vi "Client.vi"() -> ()   [LabVIEW 2018]
uses:
  <vilib>/Utility/error.llb/DialogType.ctl
  <vilib>/Utility/file.llb/Write Delimited Spreadsheet (string).vi
panel:
  in  "Address/IP":string="localhost"
  in  "Remote port or service name":u16=6340
  in  "Start":bool
  in  "file path (dialog if empty)":path=path "C:/Users/Sagar/Desktop/MEE 5318/Project4/data.txt"
  out "Waveform Graph":waveform(dbl)(graph)
  out "ai0 X-axis Waveform Graph":waveform(dbl)[](graph)
  out "ai1 Y-axis Waveform Graph":waveform(dbl)[](graph)
  out "appended array 2":dbl[][](array[numeric])
  in  "appended array":dbl[][](array[numeric])
  in  "Number of Samples":dbl=2000.0
  in  "Sample Rate":dbl=1000.0
  in  "Counter":tag="myDAQ1/ctr0"
  in  "Analog Physical Channel 1":tag="myDAQ1/ai0"
  in  "Analog Physical Channel 2":tag="myDAQ1/ai1"
  in  "IIR filter specifications":T1={"Topology"=enum."Butterworth", "Type"=enum."Lowpass", "Order"=3, "Lower Fc"=100.0, "Upper Fc"=200.0, "PB Ripple"=1.0, "SB Attenuation"=60.0} {"PB Ripple" format="%0.2f"; "SB Attenuation" format="%0.2f"; "Lower Fc" format="%0.2p"; "Upper Fc" format="%0.2p"}
  # "MEE 5318 Project 4 Client.vi\nGroup: 7\nMembers: Sagar Jagtap (903935334)\n                   Arunkumar Ramachandran (903928488)"
  # "Input following parameters and click \"START ACQUISITION\" to start acquiring data"
  # "The following graphs illustrate the acquired data"
  # "Comm Settings"
  # "Channel Settings"
  # "Timing Settings"
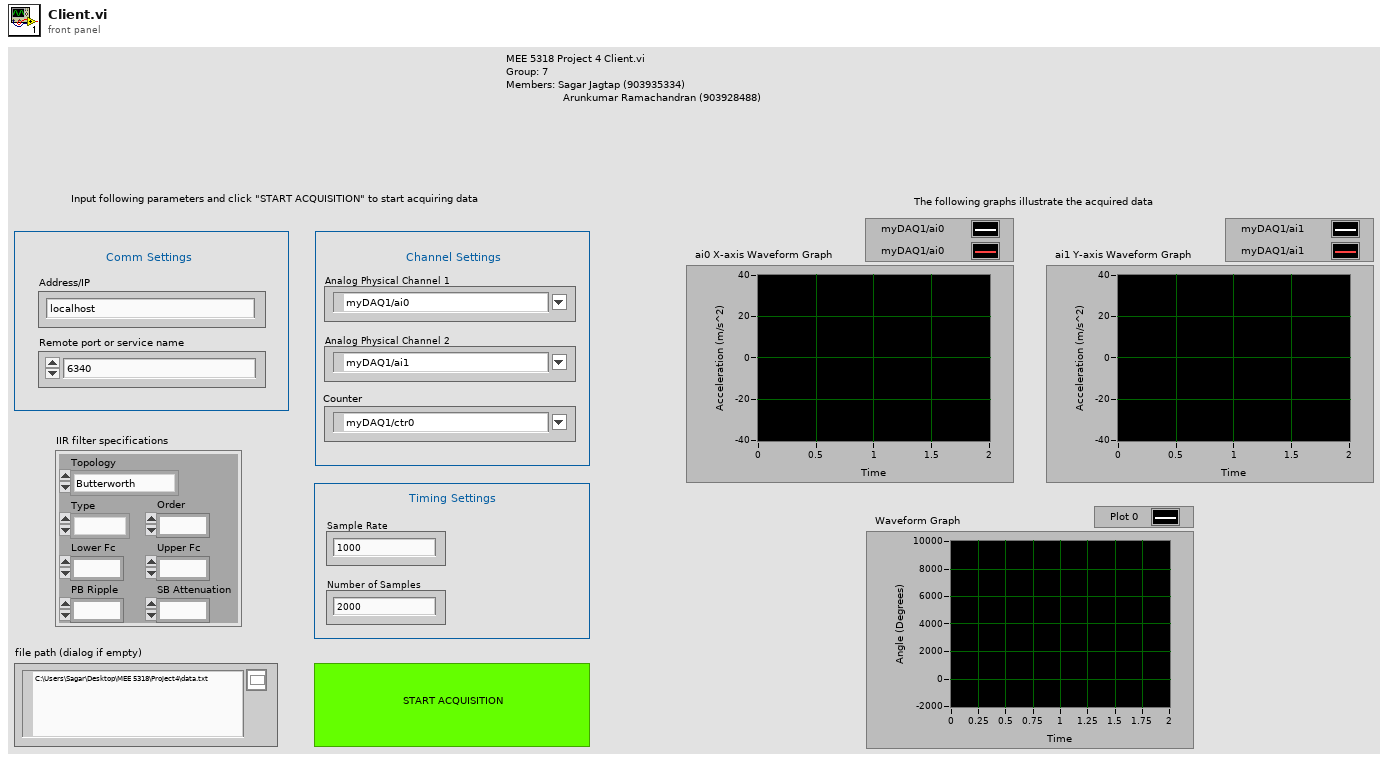
[diagram p1: front panel]
types:
  T1 = cluster{"Topology":enum16{"Off", "Butterworth", "Chebyshev", "Inverse Chebyshev", "Elliptic", "Bessel"}, "Type":enum16{"Lowpass", "Highpass", "Bandpass", "Bandstop"}, "Order":i32, "Lower Fc":dbl, "Upper Fc":dbl, "PB Ripple":dbl, "SB Attenuation":dbl}
  T2 = typedef "DialogType.ctl" = u16
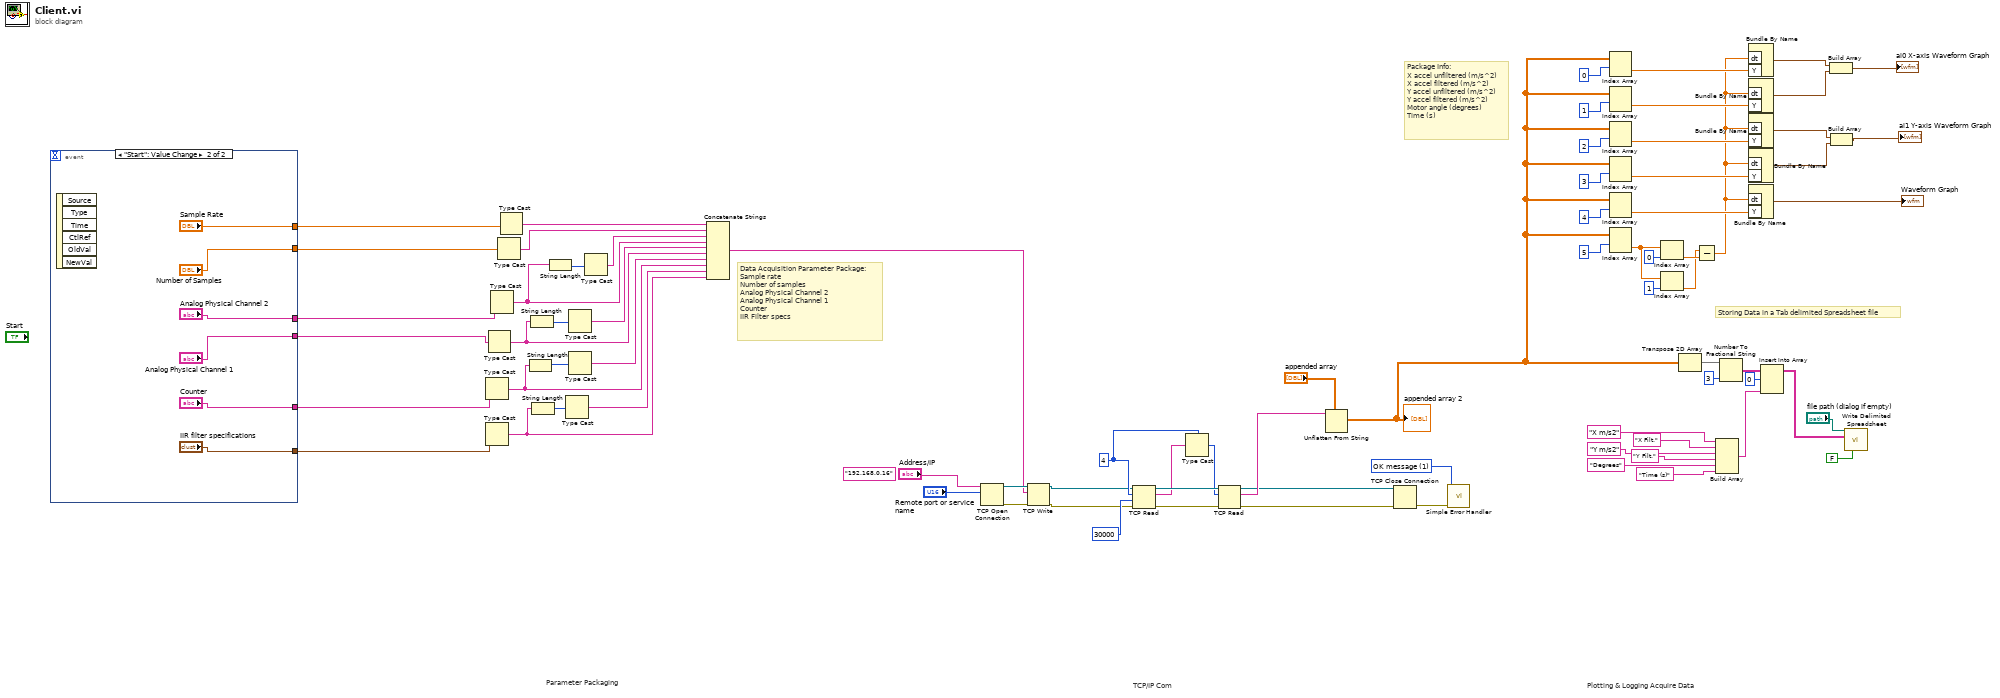
[diagram p0: block diagram]
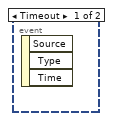
[diagram p2: hidden frame]
diagram:
  w1 = T2 1 items=["no dialog", "OK message", "continue or stop message", "OK message + warnings", "continue/stop + warnings"] ("type of dialog (OK msg:1)")
  w56 = 4 ("bytes to read")
  (unwired) "192.168.0.16" ("address")
  # "Package Info:\nX accel unfiltered (m/s^2)\nX accel filtered (m/s^2)\nY accel unfiltered (m/s^2)\nY accel filtered (m/s^2)\nMotor angle (degrees)\nTime (s)"
  # "Storing Data in a Tab delimited Spreadsheet file"
  # "Data Acquisition Parameter Package:\nSample rate\nNumber of samples\nAnalog Physical Channel 2\nAnalog Physical Channel 1\nCounter\nIIR Filter specs"
  # "Plotting & Logging Acquire Data"
  # "TCP/IP Com"
  # "Parameter Packaging"
  n1 = event shown="[1] \"Start\": Value Change" {
    selector: _ -> [_ _]
    dyn-events: _ -> [_ _]
    timeout: _ -> [_ _]
    tunnel: [_ "Number of Samples"] -> w8
    tunnel: [_ "Sample Rate"] -> w7
    tunnel: [_ "Counter"] -> w6
    tunnel: [_ "Analog Physical Channel 1"] -> w5
    tunnel: [_ "Analog Physical Channel 2"] -> w4
    tunnel: [_ "IIR filter specifications"] -> w3
    event Timeout {
      n2 = event-data() -> ()  [unwired: 1 in, 3 out]
    }
    event "Start": Value Change {
      n3 = event-data() -> ()  [unwired: 1 in, 6 out]
    }
  }
  n4 = Type Cast(x=w6) -> (*(type *) &x=w64:string)  [unwired: 1 in]
  n5 = Type Cast(x=w3) -> (*(type *) &x=w62:string)  [unwired: 1 in]
  n6 = Type Cast(x=w5) -> (*(type *) &x=w66:string)  [unwired: 1 in]
  n7 = Type Cast(x=w4) -> (*(type *) &x=w68:string)  [unwired: 1 in]
  n8 = Type Cast(x=w8) -> (*(type *) &x=w77:string)  [unwired: 1 in]
  n9 = Type Cast(x=w7) -> (*(type *) &x=w72:string)  [unwired: 1 in]
  n10 = String Length(string=w64) -> (length=w75:i32)
  n11 = String Length(string=w66) -> (length=w76:i32)
  n12 = String Length(string=w62) -> (length=w61:i32)
  n13 = String Length(string=w68) -> (length=w71:i32)
  n14 = Type Cast(x=w61) -> (*(type *) &x=w63:string)  [unwired: 1 in]
  n15 = Type Cast(x=w76) -> (*(type *) &x=w67:string)  [unwired: 1 in]
  n16 = Type Cast(x=w75) -> (*(type *) &x=w65:string)  [unwired: 1 in]
  n17 = Type Cast(x=w71) -> (*(type *) &x=w69:string)  [unwired: 1 in]
  n18 = Concatenate Strings(w72, w77, w69, w68, w67, w66, w65, w64, w63, w62) -> (w70:string)
  n19 = TCP Open Connection(address="Address/IP", remote port or service name="Remote port or service name") -> (connection ID=w74:refnum<k5>, error out=w73:errorcluster)  [unwired: 3 in]
  n20 = TCP Write(connection ID=w74, data in=w70, error in (no error)=w73) -> (connection ID out=w52:refnum<k5>, error out=w51:errorcluster)  [unwired: 1 in, 1 out]
  n21 = TCP Read(connection ID=w52, bytes to read=w56, error in (no error)=w51, 9:30000 ("timeout ms (25000)")) -> (connection ID out=w59:refnum<k5>, data out=w57:string, error out=w58:errorcluster)  [unwired: 1 in]
  n22 = Type Cast(type=w56, x=w57) -> (*(type *) &x=w55:i32)
  n23 = TCP Read(connection ID=w59, bytes to read=w55, error in (no error)=w58) -> (connection ID out=w10:refnum<k5>, data out=w54:string, error out=w9:errorcluster)  [unwired: 2 in]
  n24 = Unflatten From String(type="appended array", binary string=w54) -> (value=w29:dbl[][])  [unwired: 3 in, 2 out]
  "appended array 2" <- w29
  n25 = TCP Close Connection(connection ID=w10, error in (no error)=w9) -> (error out=w2:errorcluster)  [unwired: 1 in, 1 out]
  n26 = call <vilib>:"Simple Error Handler.vi"("type of dialog (OK msg:1)"=w1, "error in (no error)"=w2) -> ()  [unwired: 3 in, 5 out]
  n27 = Index Array(array=w29, index (row)=0) -> (element=w28:dbl[])  [unwired: 1 in]
  n28 = Index Array(array=w29, index (row)=1) -> (element=w22:dbl[])  [unwired: 1 in]
  n29 = Index Array(array=w29, index (row)=2) -> (element=w21:dbl[])  [unwired: 1 in]
  n30 = Index Array(array=w29, index (row)=3) -> (element=w20:dbl[])  [unwired: 1 in]
  n31 = Index Array(array=w29, index (row)=4) -> (element=w19:dbl[])  [unwired: 1 in]
  n32 = Index Array(array=w29, index (row)=5) -> (element=w27:dbl[])  [unwired: 1 in]
  n33 = Index Array(array=w27, index=0) -> (element=w24:dbl)
  n34 = Index Array(array=w27, index=1) -> (element=w23:dbl)
  n35 = Transpose 2D Array(2D array=w29) -> (transposed array=w49:dbl[][])
  n36 = Subtract(x=w23, y=w24) -> (x-y=w18:dbl)
  n37 = Build Array("X m/s2", "X Filt.", "Y m/s2", "Y Filt.", "Degrees", "Time (s)") -> (w47:string[])
  n38 = Number To Fractional String(number=w49, precision (6)=i16 3) -> (F-format string=w46:string[][])  [unwired: 2 in]
  n39 = Bundle By Name("dt"=w18, "Y"=w28) -> (w17:waveform(dbl))  [unwired: 1 in]
  n40 = Bundle By Name("dt"=w18, "Y"=w22) -> (w16:waveform(dbl))  [unwired: 1 in]
  n41 = Bundle By Name("dt"=w18, "Y"=w21) -> (w15:waveform(dbl))  [unwired: 1 in]
  n42 = Bundle By Name("dt"=w18, "Y"=w20) -> (w14:waveform(dbl))  [unwired: 1 in]
  n43 = Bundle By Name("dt"=w18, "Y"=w19) -> (→"Waveform Graph":waveform(dbl))  [unwired: 1 in]
  n44 = Insert Into Array(array=w46, index (row)=0, new element=w47) -> (w48:string[][])  [unwired: 1 in]
  n45 = Build Array(w17, w16) -> (→"ai0 X-axis Waveform Graph":waveform(dbl)[])
  n46 = Build Array(w15, w14) -> (→"ai1 Y-axis Waveform Graph":waveform(dbl)[])
  n47 = call-poly <vilib>:"Write Delimited Spreadsheet.vi"("file path (dialog if empty)"="file path (dialog if empty)", "2D data"=w48, "transpose? (no:F)"=FALSE) -> ()  [unwired: 11 in, 2 out]
